vi "Collect Signal on Datavalid (Multiple).vi"(5 "Input 1":dbl, 7 "Input 2":dbl, 9 "Data Valid":bool) -> (6 "Output 1":dbl[](array[numeric]) format="%.2f", 8 "Output 2":dbl[](array[numeric]) format="%.2f")   [LabVIEW 2011]
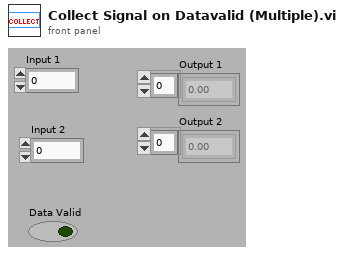
[diagram p1: front panel]
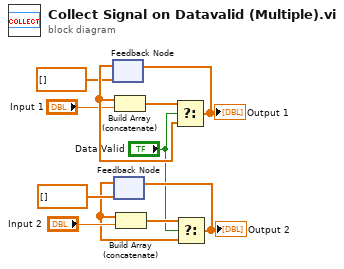
[diagram p0: block diagram]
diagram:
  n1 = feedback #1(dbl[] []) -> (w10:dbl[])
  n2 = feedback #2(dbl[] []) -> (w1:dbl[])
  n3 = Build Array (concatenate)(w10, "Input 1") -> (w7:dbl[])
  n4 = Build Array (concatenate)(w1, "Input 2") -> (w6:dbl[])
  n5 = Select(t=w7, s="Data Valid", f=w10) -> (s? t:f=w11:dbl[])
  "Output 1" <- w11
  n6 = feedback-in #1(w11) -> ()
  n7 = Select(t=w6, s="Data Valid", f=w1) -> (s? t:f=w3:dbl[])
  "Output 2" <- w3
  n8 = feedback-in #2(w3) -> ()
